vi "Close.vi"(8 "error in (no error)":errorcluster, 11 "INI Serializer in":refnum<class "INI Serializer.lvclass">) -> (0 "error out":errorcluster)   [LabVIEW 2014, in "INI Serializer.lvclass"]
uses:
  INI Serializer.lvclass
  INI Serializer.lvclass/INI Serializer.ctl
  <vilib>/Utility/config.llb/NI_LVConfig.lvlib
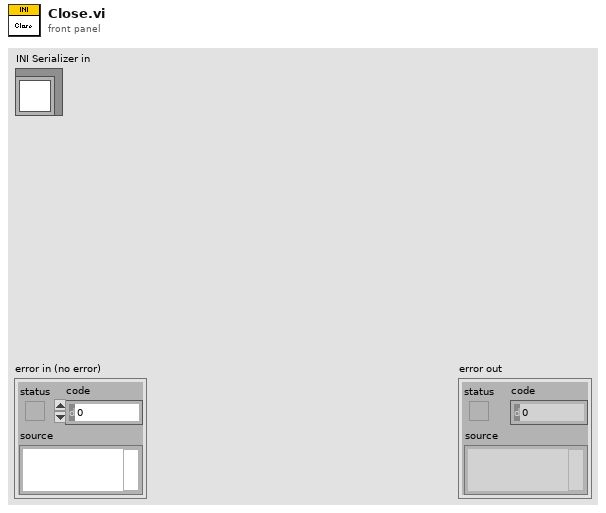
[diagram p1: front panel]
types:
  T1 = typedef "NI_LVConfig.lvlib/Config Data RefNum.ctl" = refnum<k1>
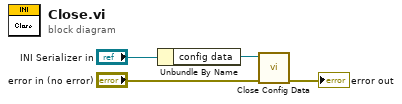
[diagram p0: block diagram]
diagram:
  n1 = Unbundle By Name("INI Serializer in") -> ("config data"=w1:T1)
  n2 = call <vilib>:"Close Config Data.vi"("error in (no error)"="error in (no error)", "refnum"=w1) -> ("error out"=→"error out":errorcluster)  [unwired: 8 in, 1 out]
